vi "Calculate Image Date.vi"(8 "error in (no error)":errorcluster, 11 "Simulated_Header in":refnum<class "Simulated_Header.lvclass">) -> (0 "error out":errorcluster, 3 "Simulated_Header out":refnum<class "Simulated_Header.lvclass">)   [LabVIEW 2018, in "Simulated_Header.lvclass"]
uses:
  Simulated_Header.lvclass
  <vilib>/Utility/miscctls.llb/LVDateTimeRec.ctl
  Simulated_Header.lvclass/Simulated_Header.ctl
panel:
  in  "date time rec":T1
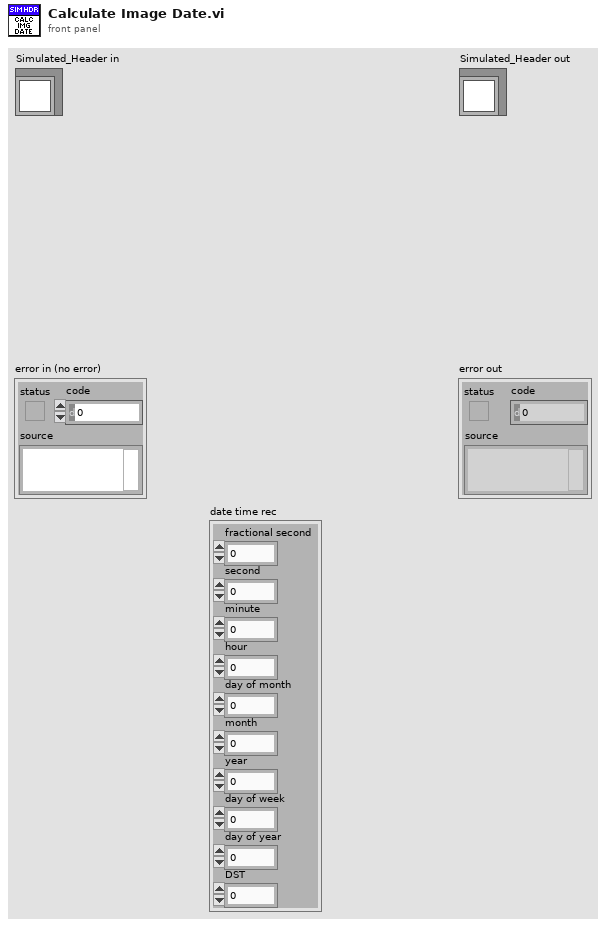
[diagram p1: front panel]
types:
  T1 = typedef "LVDateTimeRec.ctl" = cluster{"fractional second":dbl, "second":i32, "minute":i32, "hour":i32, "day of month":i32, "month":i32, "year":i32, "day of week":i32, "day of year":i32, "DST":i32}
  T2 = typedef "SYSTEMTIME structure typedef.ctl" = cluster{"Year":u16, "Month":u16, "DayOfWeek":u16, "Date":u16, "Hour":u16, "Minute":u16, "Second":u16, "Milliseconds":u16}
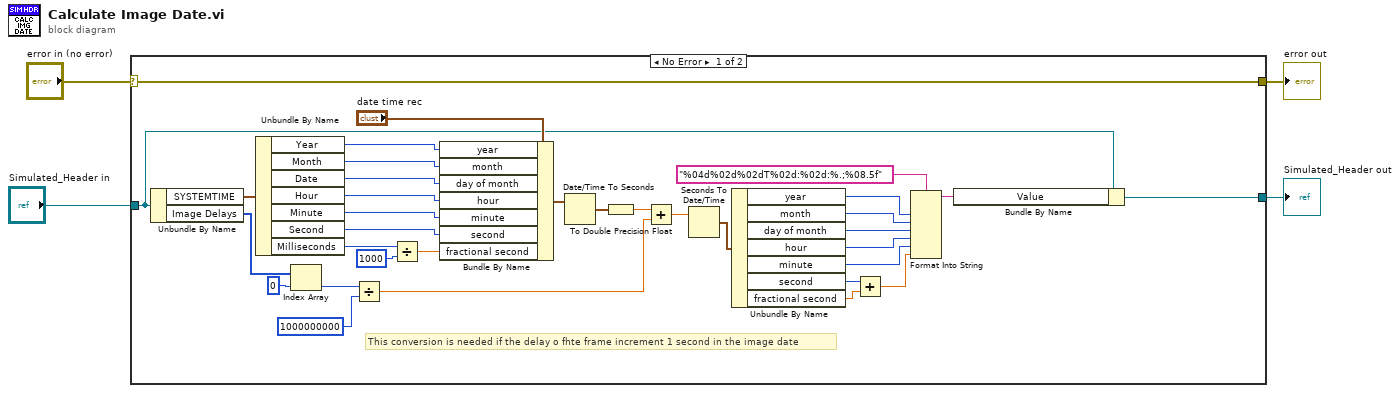
[diagram p0: block diagram]
diagram:
  n1 = case shown="No Error" "error in (no error)" {
    selector: "error in (no error)" -> [w25 w40]
    tunnel: [w25 w40] -> w3
    tunnel: [w26 w39] -> w1
    tunnel: "Simulated_Header in" -> [w27 w39]
    frame No Error {
      # "This conversion is needed if the delay o fhte frame increment 1 second in the image date"
      n2 = Unbundle By Name(w27) -> ("SYSTEMTIME"=w29:T2, "Image Delays"=w28:u32[])
      n3 = Unbundle By Name(w29) -> ("Year"=w20:u16, "Month"=w19:u16, "Date"=w18:u16, "Hour"=w17:u16, "Minute"=w16:u16, "Second"=w15:u16, "Milliseconds"=w22:u16)
      n4 = Index Array(array=w28, index=0) -> (element=w13:u32)
      n5 = Divide(x=w13, y=1000000000) -> (x/y=w32:dbl)
      n6 = Divide(x=w22, y=1000) -> (x/y=w14:dbl)
      n7 = Bundle By Name(cluster="date time rec", "year"=w20, "month"=w19, "day of month"=w18, "hour"=w17, "minute"=w16, "second"=w15, "fractional second"=w14) -> (w36:T1)
      n8 = Date/Time To Seconds(2:w36) -> (0:w35:timestamp)  [unwired: 1 in]
      n9 = To Double Precision Float(number=w35) -> (double precision float=w33:dbl)
      n10 = Add(x=w33, y=w32) -> (x+y=w31:dbl)
      n11 = Seconds To Date/Time(time stamp (now)=w31) -> (date time rec=w30:T1)  [unwired: 1 in]
      n12 = Unbundle By Name(w30) -> ("year"=w7:i32, "month"=w8:i32, "day of month"=w9:i32, "hour"=w10:i32, "minute"=w11:i32, "second"=w24:i32, "fractional second"=w23:dbl)
      n13 = Add(x=w24, y=w23) -> (x+y=w12:dbl)
      n14 = Format Into String(format string="%04d%02d%02dT%02d:%02d:%.;%08.5f", w7, w8, w9, w10, w11, w12) -> (resulting string=w6:string)  [unwired: 2 in, 1 out]
      n15 = Bundle By Name(cluster=w27, "Value"=w6) -> (w26:refnum<class "Simulated_Header.lvclass">)
    }
    frame Error {
    }
  }
  "error out" <- w3
  "Simulated_Header out" <- w1
